vi "Stop and Close SV.vi"(8 "error in (no error)":errorcluster, 11 "SV Data":T1={"Status notifier"=refnum, "Write FIFO ref"=refnum, "Read FIFO ref"=refnum, "Status FIFO ref"=refnum, "Update Rate"=1, "Write Refs by Type"={"DBL Write"=[]}, "Read Refs by Type"={"DBL Read"=[]}, "WriteSize"=0, "ReadSize"=0}) -> (0 "error out":errorcluster, 3 "SV Data":T1={"Status notifier"=refnum, "Write FIFO ref"=refnum, "Read FIFO ref"=refnum, "Status FIFO ref"=refnum, "Update Rate"=1, "Write Refs by Type"={"DBL Write"=[]}, "Read Refs by Type"={"DBL Read"=[]}, "WriteSize"=0, "ReadSize"=0})   [LabVIEW 2020, in "Shared Variable Interface.lvlib"]
uses:
  Shared Variable Interface.lvlib
  SV Process Configuration.ctl
  DataTypes/DBL.lvlib
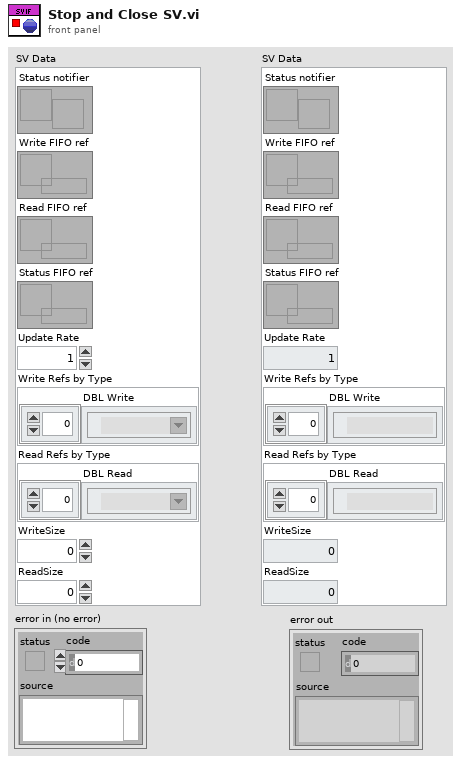
[diagram p1: front panel]
types:
  T1 = typedef "Shared Variable Interface.lvlib/SV Process Configuration.ctl" = cluster{"Status notifier":refnum<notifier>, "Write FIFO ref":refnum<k33>, "Read FIFO ref":refnum<k33>, "Status FIFO ref":refnum<k33>, "Update Rate":u32, "Write Refs by Type":cluster{"DBL Write":refnum<k21>[]}, "Read Refs by Type":cluster{"DBL Read":refnum<k21>[]}, "WriteSize":i32, "ReadSize":i32}
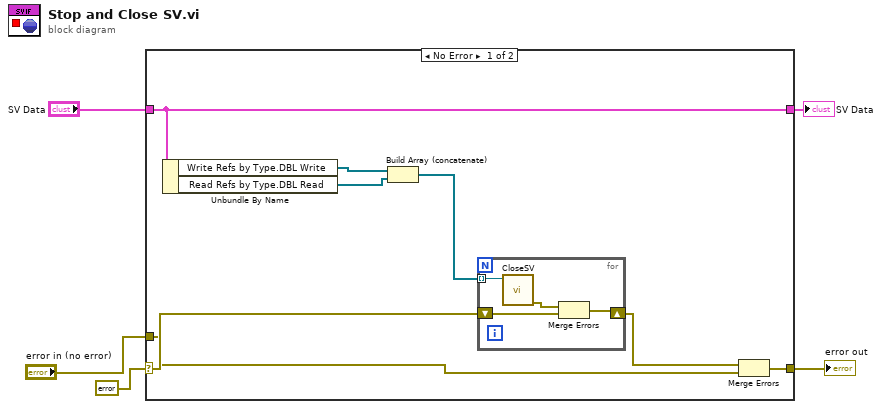
[diagram p0: block diagram]
diagram:
  n1 = case shown="No Error" errorcluster {"status"=FALSE, "code"=0, "source"=""} ("error IO") {
    selector: errorcluster {"status"=FALSE, "code"=0, "source"=""} ("error IO") -> [w10 w19]
    tunnel: [w13 w19] -> w5
    tunnel: "error in (no error)" -> [w9 _]
    tunnel: "SV Data" -> [w6 w18]
    tunnel: [w6 w18] -> w1
    frame No Error {
      n2 = Unbundle By Name(w6) -> ("Write Refs by Type.DBL Write"=w8:refnum<k21>[], "Read Refs by Type.DBL Read"=w7:refnum<k21>[])
      n3 = Build Array (concatenate)(w8, w7) -> (w12:refnum<k21>[])
      n4 = for {
        shift-right: [w16] -> w11
        shift-left: w10 -> [w17]
        tunnel: w12 -> [w14] mode=indexing
        n5 = call "CloseSV.vi"("Shared variable refnum"=w14) -> ("error out"=w15:errorcluster)  [unwired: 10 in]
        n6 = Merge Errors(w15, w17) -> (w16:errorcluster)
      }
      n7 = Merge Errors(w11, w9) -> (w13:errorcluster)
    }
    frame Error {
    }
  }
  "error out" <- w5
  "SV Data" <- w1
